vi "Query Grating.vi"(8 "error in (no error)":errorcluster, 11 "VISA resource name":refnum<visa-resource-name>) -> (0 "error out":errorcluster, 1 "BLAZE (nm)":u16 step=1, 2 "GRATING #":u8, 3 "VISA resource name out":refnum<visa-resource-name>, 4 "GR/MM":u16 step=1, 5 "# OF GRATINGS":u8 max=3 step=1)   [LabVIEW 2015, in "Digikrom DK24x.lvlib"]
doc: "Returns the current grating ruling identifier."
uses:
  Digikrom DK24x.lvlib
  Private/Command.ctl
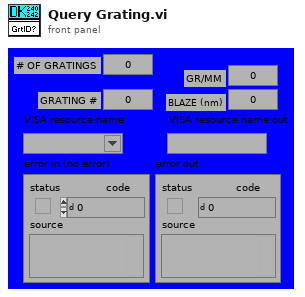
[diagram p1: front panel]
types:
  T1 = typedef "Digikrom DK24x.lvlib/Command.ctl" = u8
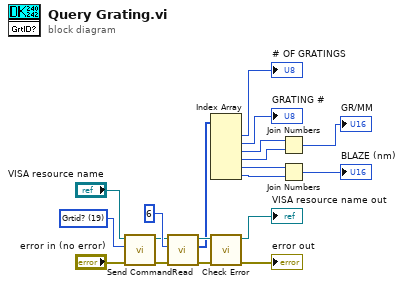
[diagram p0: block diagram]
diagram:
  w1 = T1 19 items=["Cancel"=24, "Clear"=25, "CSR"=28, "Echo"=27, "Filter"=15, "Gcal"=18, "Goto"=16, "Grtid?"=19, "Grtsel"=26, "NOVRAM Read"=56, "NOVRAM Write"=59, "Reset"=255, "Scan"=12, "Scan Up"=9, "Scan Down"=3, "Serial?"=33, "Slew Up"=8, "Slew Down"=2, "Slit Reset"=43, "Slit?"=30, "Sltadj"=14, "Speed"=13, "Sspeed?"=21, "Step Down"=1, "Step Up"=7, "S1adj"=31, "S2adj"=32, "S3adj"=34, "S1cal"=22, "S2cal"=23, "S3cal"=35, "Test"=17, "Type"=57, "Wave?"=29, "Zero"=52] ("Command")
  n1 = call "Send Command.vi"("error in (no error)"="error in (no error)", "Command"=w1, "VISA resource name"="VISA resource name") -> ("error out"=w16:errorcluster, "VISA resource name out"=w15:refnum<visa-resource-name>)  [unwired: 7 out]
  n2 = call "Read.vi"("error in (no error)"=w16, "response size"=u8 6, "VISA resource name"=w15) -> ("error out"=w12:errorcluster, "response array"=w8:u8[], "VISA resource name out"=w11:refnum<visa-resource-name>)  [unwired: 6 out]
  n3 = Index Array(array=w8) -> (element #1=→"# OF GRATINGS":u8, element #2=→"GRATING #":u8, element #3=w5:u8, element #4=w4:u8, element #5=w3:u8, element #6=w2:u8)  [unwired: 6 in]
  n4 = call "Check Error.vi"("error in"=w12, "VISA resource name in"=w11) -> ("error out"=→"error out":errorcluster, "VISA resource name out"=→"VISA resource name out":refnum<visa-resource-name>)  [unwired: 1 in, 7 out]
  n5 = Join Numbers(hi=w5, lo=w4) -> ((hi.lo)=→"GR/MM":u16)
  n6 = Join Numbers(hi=w3, lo=w2) -> ((hi.lo)=→"BLAZE (nm)":u16)
